vi "Clamp_Main Function.vi"(0 "Refnum in":T3, 2 "Clamp Settings":T4, 3 "ROI":T5, 5 "error in (no error)":errorcluster, 8 "Process In":u16(ring)) -> (7 "Line Coordinates":T1(array[cluster]) {"?"."Y" format="%.2f"; "?"."X" format="%.2f"; "?"."Y" format="%.2f"; "?"."X" format="%.2f"}, 9 "appended array":cluster{"X":sgl, "Y":sgl}[](array[cluster]), 11 "Perpendicular Lines":T1(array[cluster]), 13 "Points":cluster{"X":sgl, "Y":sgl}[](array[cluster]), 14 "Refnum out":T3, 16 "Distance":sgl, 17 "Edge Coordinates":cluster{"X":sgl, "Y":sgl}[](array[cluster]) {"Y" format="%.2f"; "X" format="%.2f"}, 19 "error out":errorcluster)   [LabVIEW 2019]
uses:
  <vilib>/vision/Image Controls.llb/IMAQ Image.ctl
panel:
  out "Coordinate System (duplicate)":T2 {"Measurement System"."Axis Reference" items=["Direct", "Indirect"]; "Measurement System"."Angle (deg)" format="%.2f"; "Measurement System"."Origin"."Y" format="%.2f"; "Measurement System"."Origin"."X" format="%.2f"; "Reference System"."Axis Reference" items=["Direct", "Indirect"]; "Reference System"."Angle (deg)" format="%.2f"; "Reference System"."Origin"."Y" format="%.2f"; "Reference System"."Origin"."X" format="%.2f"}
  # "Start Point"
  # "End Point"
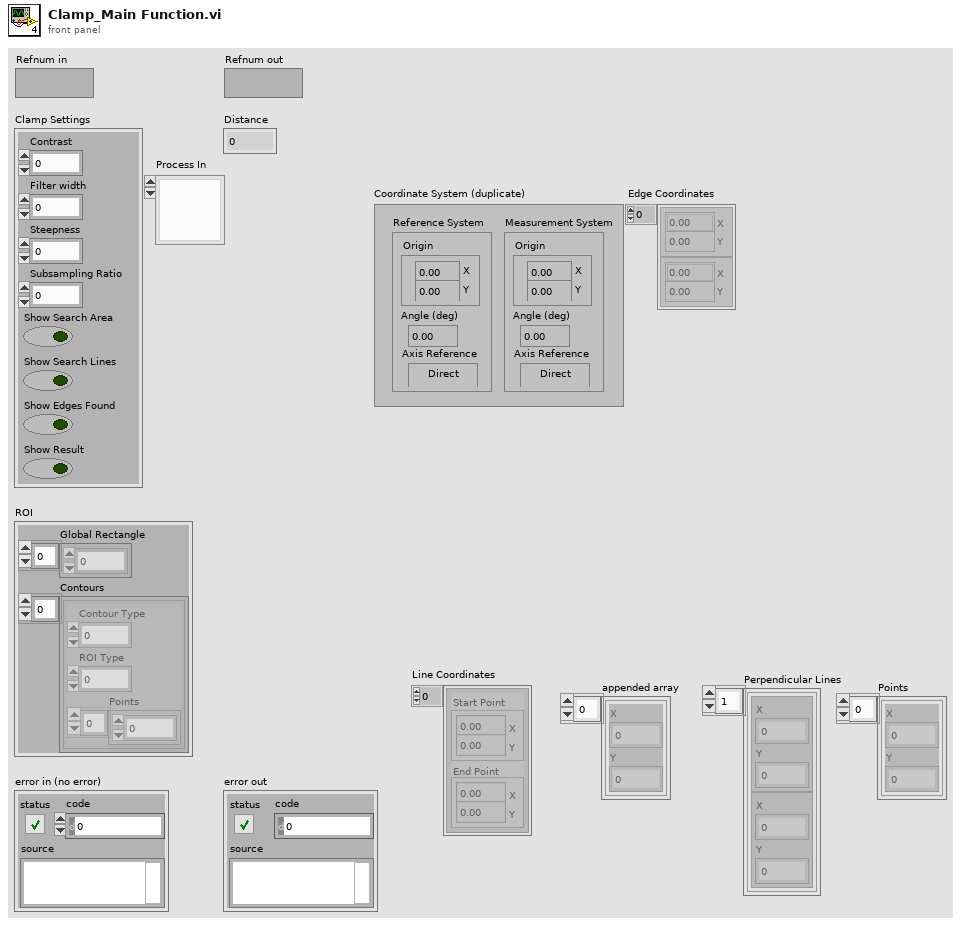
[diagram p1: front panel]
types:
  T1 = cluster{cluster{"X":sgl, "Y":sgl}, cluster{"X":sgl, "Y":sgl}}[]
  T2 = typedef "IMAQ Coordinate System" = cluster{"Reference System":cluster{"Origin":cluster{"X":sgl, "Y":sgl}, "Angle (deg)":sgl, "Axis Reference":u32}, "Measurement System":cluster{"Origin":cluster{"X":sgl, "Y":sgl}, "Angle (deg)":sgl, "Axis Reference":u32}}
  T3 = typedef "IMAQ Image.ctl" = refnum<image>
  T4 = cluster{"Contrast":i32, "Filter width":i32, "Steepness":i32, "Subsampling Ratio":u32, "Show Search Area":bool, "Show Search Lines":bool, "Show Edges Found":bool, "Show Result":bool}
  T5 = cluster{"Global Rectangle":i32[], "Contours":cluster{"Contour Type":u32, "ROI Type":u32, "Points":i32[]}[]}
  T6 = typedef "IMAQ Rectangle" = cluster{"Left":i32, "Top":i32, "Right":i32, "Bottom":i32, "Rotation":dbl}
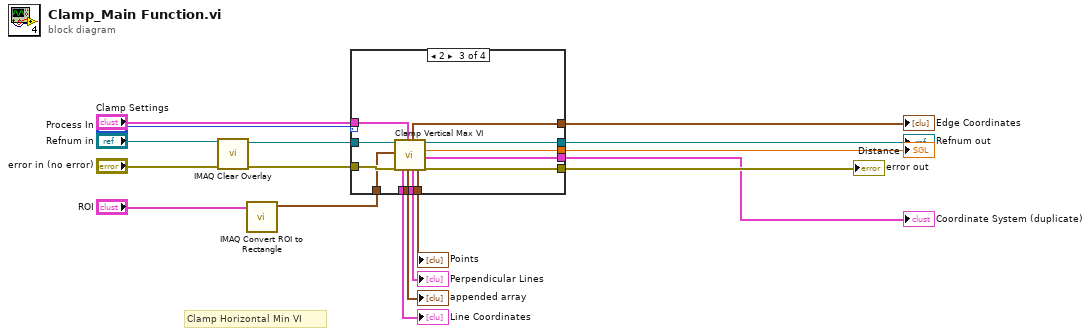
[diagram p0: block diagram]
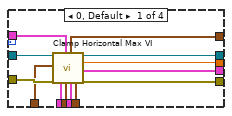
[diagram p2: hidden frame]
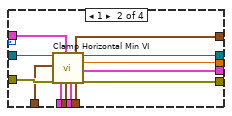
[diagram p3: hidden frame]
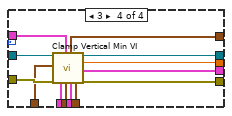
[diagram p4: hidden frame]
diagram:
  # "Clamp Horizontal Min VI"
  n1 = call "IMAQ Clear Overlay"("error in (no error)"="error in (no error)", "Image"="Refnum in") -> ("error out"=w7:errorcluster, "Image Out"=w8:T3)  [unwired: 8 in]
  n2 = call "IMAQ Convert ROI to Rectangle"("ROI Descriptor"="ROI") -> ("Rectangle"=w5:T6)  [unwired: 8 in, 1 out]
  n3 = case shown="2" "Process In" {
    tunnel: w7 -> [w30 w42 w55 w68]
    tunnel: w8 -> [w29 w41 w54 w67]
    tunnel: [w28 w40 w53 w66] -> w17
    tunnel: "Clamp Settings" -> [w22 w39 w52 w65]
    tunnel: [w27 w38 w51 w64] -> w15
    tunnel: [w26 w37 w50 w63] -> w13
    tunnel: [w25 w36 w49 w62] -> w11
    tunnel: [w24 w31 w48 w61] -> w10
    tunnel: w5 -> [w23 w35 w47 w60]
    tunnel: [w21 w34 w46 w59] -> w4
    tunnel: [w20 w33 w45 w58] -> w3
    tunnel: [w19 w32 w44 w57] -> w2
    tunnel: [w18 w31 w43 w56] -> w1
    frame 0, Default {
      n4 = call "Clamp Horizontal Max VI.vi"("Image"=w29, "Rectangle"=w23, "error in (no error)"=w30, "Settings"=w22) -> ("Line Coordinates"=w21:T1, "appended array"=w20:cluster{"X":sgl, "Y":sgl}[], "Edge Coordinates"=w24:cluster{"X":sgl, "Y":sgl}[], "Perpendicular Lines"=w19:T1, "Points"=w18:cluster{"X":sgl, "Y":sgl}[], "Image Out"=w26:T3, "Distance"=w28:sgl, "Coordinate System (duplicate)"=w25:T2, "error out"=w27:errorcluster)  [unwired: 7 in]
    }
    frame 1 {
      n5 = call "Clamp Horizontal Min VI.vi"("Image"=w41, "Rectangle"=w35, "error in (no error)"=w42, "Settings"=w39) -> ("Line Coordinates"=w34:T1, "appended array"=w33:cluster{"X":sgl, "Y":sgl}[], "Perpendicular Lines"=w32:T1, "Points"=w31:cluster{"X":sgl, "Y":sgl}[], "Image Out"=w37:T3, "Distance"=w40:sgl, "Coordinate System (duplicate)"=w36:T2, "error out"=w38:errorcluster)  [unwired: 8 in]
    }
    frame 2 {
      n6 = call "Clamp Vertical Max VI.vi"("Image"=w54, "Rectangle"=w47, "error in (no error)"=w55, "Settings"=w52) -> ("Line Coordinates"=w46:T1, "appended array"=w45:cluster{"X":sgl, "Y":sgl}[], "Edge Coordinates"=w48:cluster{"X":sgl, "Y":sgl}[], "Perpendicular Lines"=w44:T1, "Points"=w43:cluster{"X":sgl, "Y":sgl}[], "Image Out"=w50:T3, "Distance"=w53:sgl, "Coordinate System (duplicate)"=w49:T2, "error out"=w51:errorcluster)  [unwired: 7 in]
    }
    frame 3 {
      n7 = call "Clamp Vertical Min VI.vi"("Image"=w67, "Rectangle"=w60, "error in (no error)"=w68, "Settings"=w65) -> ("Line Coordinates"=w59:T1, "appended array"=w58:cluster{"X":sgl, "Y":sgl}[], "Edge Coordinates"=w61:cluster{"X":sgl, "Y":sgl}[], "Perpendicular Lines"=w57:T1, "Points"=w56:cluster{"X":sgl, "Y":sgl}[], "Image Out"=w63:T3, "Distance"=w66:sgl, "Coordinate System (duplicate)"=w62:T2, "error out"=w64:errorcluster)  [unwired: 7 in]
    }
  }
  "Distance" <- w17
  "error out" <- w15
  "Refnum out" <- w13
  "Coordinate System (duplicate)" <- w11
  "Edge Coordinates" <- w10
  "Line Coordinates" <- w4
  "appended array" <- w3
  "Perpendicular Lines" <- w2
  "Points" <- w1
